vi "From JSON.vi"(8 "error in (no error)":errorcluster, 10 "JSON":string) -> (0 "error out":errorcluster, 3 "ConfigInfoValue out":refnum<class "ConfigInfoValue.lvclass">)   [LabVIEW 2020, in "Volatus.lvlib" / "ConfigInfoValue.lvclass"]
uses:
  ConfigInfoValue.lvclass
  ConfigInfoValue.lvclass/ConfigInfoValue.ctl
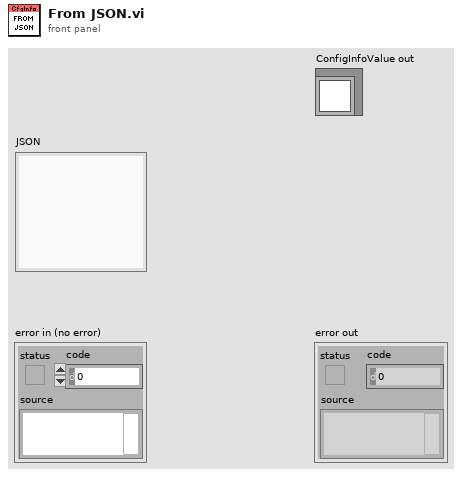
[diagram p1: front panel]
types:
  T1 = cluster{"System":string, "Cluster":string, "Node":string, "Path":string, "Version":string, "Hash":string}
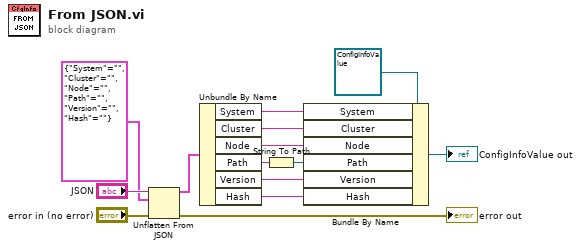
[diagram p0: block diagram]
diagram:
  n1 = Unflatten From JSON(JSON string="JSON", type and defaults=T1 {"System"="", "Cluster"="", "Node"="", "Path"="", "Version"="", "Hash"=""} ("cluster"), error in (no error)="error in (no error)") -> (value=w9:T1, error out=→"error out":errorcluster)  [unwired: 4 in]
  n2 = Unbundle By Name(w9) -> ("System"=w7:string, "Cluster"=w6:string, "Node"=w5:string, "Path"=w2:string, "Version"=w4:string, "Hash"=w3:string)
  n3 = String To Path(string=w2) -> (path=w1:path)
  n4 = Bundle By Name(cluster=refnum<class "ConfigInfoValue.lvclass"> refnum ("ConfigInfoValue in"), "System"=w7, "Cluster"=w6, "Node"=w5, "Path"=w1, "Version"=w4, "Hash"=w3) -> (→"ConfigInfoValue out":refnum<class "ConfigInfoValue.lvclass">)
